vi "HFRR ADV v025 new software.vi"() -> ()   [LabVIEW 2025] (continued)
            n902 = call <vilib>:"Trim Whitespace.vi"("string"="C:\\LAB-IQ\\images\\") -> ("trimmed string"=w1151:string)  [unwired: 1 in]
            n903 = String To Path(string=w1151) -> (path=w1150:path)
            n904 = Concatenate Strings(w1149, ".png" ("string")) -> (w1148:string)
            n905 = Build Path(base path=w1150, name or relative path=w1148) -> (appended path=w1146:path)
            n906 = Path To String(path=w1146) -> (string=w1145:string)
            n907 = call "CAMERA LIVE FEED FGV.vi"("Enum - Menu"=CAMERA_LIVE_FEED_ENUM."CAMERA SAVE", "Image Path"=w1145) -> ("error out"=w1143:errorcluster)  [unwired: 8 in, 1 out]
            n908 = case shown="No Error" w1143 {
              frame No Error {
                n909 = One Button Dialog(message="Image saved successfully") -> ()  [unwired: 1 in, 1 out]
              }
              frame Error {
              }
            }
          }
          frame #3 {
            n910 = call "LIST FILE NAMES.vi"() -> ("error out"=w1157:errorcluster, "filenames"=w1154:string[])  [unwired: 10 in]
            n911 = call "IMAGE ANALYSIS.vi"("Enum"=POST_ANALYSIS_ENUM."SHOW UI", "error in"=w1157) -> ("error out"=w1155:errorcluster)  [unwired: 8 in, 1 out]
            n912 = property on="Test File List :" class="CmbBox"("Strings[]"=w1154) -> ()  [unwired: 2 in, 2 out]
          }
          frame #4 {
            (unwired) T22."Report" ("Main Dashboard Buttons")
            (unwired) T24."Report" ("Main Dashboard Buttons")
            n913 = Not(x=w1162) -> (.not. x?=w1161:bool)
            n914 = local write "Zoom Factore"(0.0 ("Zoom Factore")) -> ()
            n915 = local write "Cap Live Image"(w1161) -> ()
            n916 = local write "Main Tab"(T2."Adv Scar Report" ("Main Tab")) -> ()
            n917 = property on="Cap Live Image" class="Bool (strict)"("BoolText.Text"="Capture Image" ("Boolean Text.Text")) -> ()  [unwired: 2 in, 2 out]
            n918 = local write "Main Dashboard Buttons"(T1."Report" ("Main Dashboard Buttons")) -> ()
          }
        }
      }
    }
    n919 = local read "change Gain"() -> (w808:bool)
    n920 = local read "Back Square"() -> (w807:bool)
    n921 = case shown="True" w808 {
      selector: w808 -> [_ w852]
      frame False {
      }
      frame True {
        n922 = stacked-sequence {
          tunnel: w852 -> [_ w860]
          frame #0 {
            n923 = local read "Actual (µm)"() -> (w856:dbl)
            n924 = local read "Pixel Value"() -> (w855:dbl)
            n925 = local read "Magnification :"() -> (w854:string)
            n926 = Divide(x=w856, y=w855) -> (x/y=w853:dbl)
            n927 = case shown="\"10x\"" w854 {
              tunnel: w853 -> [w857 w858]
              frame "10x" {
                n928 = local write "10x Gain"(w857) -> ()
              }
              frame "5x", Default {
                n929 = local write "5x Gain"(w858) -> ()
              }
            }
          }
          frame #1 {
            n930 = Not(x=w860) -> (.not. x?=w859:bool)
            n931 = local write "change Gain"(w859) -> ()
          }
        }
      }
    }
    n932 = case shown="True" w807 {
      selector: w807 -> [_ w850]
      frame False {
      }
      frame True {
        n933 = Not(x=w850) -> (.not. x?=w849:bool)
        n934 = local write "Back Square"(w849) -> ()
        n935 = local write "Calibration Tab"(enum32{"Measrument", "Calibrate"}."Measrument" ("Calibration Tab")) -> ()
      }
    }
    n936 = local read "Rectangle Tool"() -> (w819:bool)
    n937 = local read "Clear ROI Tool"() -> (w818:bool)
    n938 = local read "Open Image"() -> (w823:bool)
    n939 = local read "line tool"() -> (w820:bool)
    n940 = local read "OUT"() -> (w821:bool)
    n941 = local read "In"() -> (w822:bool)
    n942 = case shown="True" w823 {
      selector: w823 -> [_ w1128]
      tunnel: [w1124 w1130] -> _
      tunnel: w813 -> [w1124 w1129]
      frame False {
      }
      frame True {
        n943 = Not(x=w1128) -> (.not. x?=w1127:bool)
        n944 = local write "Open Image"(w1127) -> ()
        n945 = call "IMAGE ANALYSIS.vi"("Enum"=POST_ANALYSIS_ENUM."HIDE UI", "error in"=w1129) -> ("error out"=w1137:errorcluster)  [unwired: 8 in, 1 out]
        n946 = call "File Dialog"("start path"=path "C:/LAB-IQ/images", "error in"=w1137) -> ("selected path"=w1126:path, "error out"=w1135:errorcluster)  [unwired: 10 in, 2 out]
        "Image path  2" <- w1126
        n947 = call <vilib>:"Clear Errors.vi"("error in (no error)"=w1135) -> ("error out"=w1134:errorcluster)  [unwired: 5 in, 1 out]
        n948 = call "IMAGE ANALYSIS.vi"("Enum"=POST_ANALYSIS_ENUM."OPEN FILE", "error in"=w1134, "File Path"=w1126) -> ("error out"=w1133:errorcluster)  [unwired: 7 in, 1 out]
        n949 = call <vilib>:"Clear Errors.vi"("error in (no error)"=w1133) -> ("error out"=w1132:errorcluster)  [unwired: 5 in, 1 out]
        n950 = call "IMAGE ANALYSIS.vi"("Enum"=POST_ANALYSIS_ENUM."SHOW UI", "error in"=w1132) -> ("error out"=w1130:errorcluster)  [unwired: 8 in, 1 out]
        n951 = local write "Zoom Factore"(100.0 ("Zoom Factore")) -> ()
      }
    }
    n952 = case shown="True" w821 {
      selector: w821 -> [_ w1109]
      tunnel: w813 -> [w1106 w1114]
      tunnel: [w1106 w1108] -> _
      frame False {
      }
      frame True {
        n953 = Not(x=w1109) -> (.not. x?=w1107:bool)
        n954 = local read "Zoom Factore"() -> (w1112:dbl)
        n955 = local write "OUT"(w1107) -> ()
        n956 = call "IMAGE ANALYSIS.vi"("Enum"=POST_ANALYSIS_ENUM."ZOOM OUT", "error in"=w1114) -> ("error out"=w1108:errorcluster)  [unwired: 8 in, 1 out]
        n957 = Divide(x=w1112, y=1.2) -> (x/y=w1110:dbl)
        n958 = local write "Zoom Factore"(w1110) -> ()
      }
    }
    n959 = case shown="True" w822 {
      selector: w822 -> [_ w1118]
      tunnel: w813 -> [w1115 w1123]
      tunnel: [w1115 w1116] -> _
      frame False {
      }
      frame True {
        n960 = Not(x=w1118) -> (.not. x?=w1117:bool)
        n961 = local read "Zoom Factore"() -> (w1121:dbl)
        n962 = local write "In"(w1117) -> ()
        n963 = call "IMAGE ANALYSIS.vi"("Enum"=POST_ANALYSIS_ENUM."ZOOM IN", "error in"=w1123) -> ("error out"=w1116:errorcluster)  [unwired: 8 in, 1 out]
        n964 = Multiply(x=w1121, y=1.2) -> (x*y=w1119:dbl)
        n965 = local write "Zoom Factore"(w1119) -> ()
      }
    }
    n966 = case shown="True" w818 {
      selector: w818 -> [_ w1090]
      tunnel: w813 -> [w1088 w1092]
      tunnel: [w1088 w1091] -> _
      frame False {
      }
      frame True {
        n967 = Not(x=w1090) -> (.not. x?=w1089:bool)
        n968 = local write "Clear ROI Tool"(w1089) -> ()
        n969 = call "IMAGE ANALYSIS.vi"("Enum"=POST_ANALYSIS_ENUM."CLEAR ROI", "error in"=w1092) -> ("error out"=w1091:errorcluster)  [unwired: 8 in, 1 out]
      }
    }
    n970 = case shown="True" w820 {
      selector: w820 -> [_ w1102]
      tunnel: w813 -> [w1100 w1105]
      tunnel: [w1100 w1103] -> _
      frame False {
      }
      frame True {
        n971 = Not(x=w1102) -> (.not. x?=w1101:bool)
        n972 = local write "line tool"(w1101) -> ()
        n973 = call "IMAGE ANALYSIS.vi"("Enum"=POST_ANALYSIS_ENUM."DRAW LINE", "error in"=w1105) -> ("error out"=w1103:errorcluster)  [unwired: 8 in, 1 out]
      }
    }
    n974 = case shown="True" w819 {
      selector: w819 -> [_ w1096]
      tunnel: w813 -> [w1094 w1098]
      tunnel: [w1094 w1097] -> _
      frame False {
      }
      frame True {
        n975 = Not(x=w1096) -> (.not. x?=w1095:bool)
        n976 = local write "Rectangle Tool"(w1095) -> ()
        n977 = call "IMAGE ANALYSIS.vi"("Enum"=POST_ANALYSIS_ENUM."DRAW REC", "error in"=w1098) -> ("error out"=w1097:errorcluster)  [unwired: 8 in, 1 out]
      }
    }
    n978 = local read "SCAR MEASURMENT"() -> (w806:enum32{"Auto Scar", "Manual Scar"})
    n979 = local read "Fit to Screen Tool"() -> (w815:bool)
    n980 = local read "Resize Tool"() -> (w814:bool)
    n981 = case shown="\"Manual Scar\", Default" w806 {
      frame "Auto Scar" {
        n982 = property on="Cap Live Image" class="Bool (strict)"("BoolText.Text"="Report" ("Boolean Text.Text")) -> ()  [unwired: 2 in, 2 out]
      }
      frame "Manual Scar", Default {
        n983 = property on="Cap Live Image" class="Bool (strict)"("BoolText.Text"="Save Image" ("Boolean Text.Text")) -> ()  [unwired: 2 in, 2 out]
      }
    }
    n984 = local read "ROI Color Tool"() -> (w816:bool)
    n985 = local read "Pan Tool"() -> (w817:bool)
    n986 = case shown="True" w817 {
      selector: w817 -> [_ w1084]
      tunnel: w813 -> [w1082 w1086]
      tunnel: [w1082 w1085] -> _
      frame False {
      }
      frame True {
        n987 = Not(x=w1084) -> (.not. x?=w1083:bool)
        n988 = call "IMAGE ANALYSIS.vi"("Enum"=POST_ANALYSIS_ENUM."PAN", "error in"=w1086) -> ("error out"=w1085:errorcluster)  [unwired: 8 in, 1 out]
        n989 = local write "Pan Tool"(w1083) -> ()
      }
    }
    n990 = case shown="True" w814 {
      selector: w814 -> [_ w1068]
      tunnel: w813 -> [w1063 w1065]
      tunnel: [w1063 w1064] -> _
      frame False {
      }
      frame True {
        n991 = Not(x=w1068) -> (.not. x?=w1067:bool)
        n992 = local write "Resize Tool"(w1067) -> ()
        n993 = call "IMAGE ANALYSIS.vi"("Enum"=POST_ANALYSIS_ENUM."RESIZE MODE", "error in"=w1065) -> ("error out"=w1064:errorcluster)  [unwired: 8 in, 1 out]
      }
    }
    n994 = case shown="True" w815 {
      selector: w815 -> [_ w1073]
      tunnel: [w1069 w1074] -> _
      tunnel: w813 -> [w1069 w1072]
      frame False {
      }
      frame True {
        n995 = Not(x=w1073) -> (.not. x?=w1071:bool)
        n996 = local write "Zoom Factore"(100.0 ("Zoom Factore")) -> ()
        n997 = local write "Fit to Screen Tool"(w1071) -> ()
        n998 = call "IMAGE ANALYSIS.vi"("Enum"=POST_ANALYSIS_ENUM."FIT", "error in"=w1072) -> ("error out"=w1074:errorcluster)  [unwired: 8 in, 1 out]
      }
    }
    n999 = case shown="True" w816 {
      selector: w816 -> [_ w1079]
      tunnel: [w1076 w1080] -> _
      tunnel: w813 -> [w1076 w1077]
      frame False {
      }
      frame True {
        n1000 = Not(x=w1079) -> (.not. x?=w1078:bool)
        n1001 = local write "ROI Color Tool"(w1078) -> ()
        n1002 = call "IMAGE ANALYSIS.vi"("Enum"=POST_ANALYSIS_ENUM."SET ROI COLOR", "error in"=w1077) -> ("error out"=w1080:errorcluster)  [unwired: 8 in, 1 out]
      }
    }
    n1003 = local read "Quit"() -> (w830:bool)
  }
  n1004 = while {
    stop <- w1164 stop-if-true
    n1005 = local read "Image Path"() -> (w1167:path)
    n1006 = local read "Print 3"() -> (w1170:bool)
    n1007 = Equal?(x=w1167, y=path "") -> (x = y?=w1166:bool)
    n1008 = Not(x=w1166) -> (.not. x?=w1165:bool)
    n1009 = property on="Print 3" class="Bool (strict)"("Visible"=w1165) -> ()  [unwired: 2 in, 2 out]
    n1010 = case shown="True" w1170 {
      frame False {
        n1011 = local write "Rd"(TRUE ("Boolean 7")) -> ()
      }
      frame True {
        n1012 = flat-sequence {
          tunnel: [w1210] -> w1178
          tunnel: [w1197] -> w1176
          tunnel: [w1207] -> w1172
          tunnel: w1178 -> [w1219]
          tunnel: [w1219] -> w1177
          tunnel: w1176 -> [w1218]
          tunnel: [w1218] -> w1175
          tunnel: [w1216] -> w1174
          tunnel: [w1215] -> w1173
          tunnel: w1172 -> [w1215]
          tunnel: w1177 -> [w1221]
          tunnel: w1175 -> [w1222]
          tunnel: w1174 -> [_]
          tunnel: w1173 -> [w1220]
          frame #0 {
            n1013 = case shown="True" "Rd" {
              frame False {
              }
              frame True {
                n1014 = while {
                  tunnel: "abcdefABCDEF" ("string 2") -> [w1189]
                  shift-right: [w1187] -> w1181
                  shift-left: "" -> [w1186]
                  i -> [w1196]
                  stop <- w1195 stop-if-true
                  n1015 = Random Number (0-1)() -> (number: 0 to 1=w1190:dbl)
                  n1016 = Multiply(x=w1190, y=62.0) -> (x*y=w1192:dbl)
                  n1017 = Decrement(x="Length 2") -> (x-1=w1185:i16)
                  n1018 = To Word Integer(number=w1192) -> (16bit integer=w1193:i16)
                  n1019 = String Subset(string=w1189, offset (0)=w1193, length (rest)=1 ("length (rest)")) -> (substring=w1188:string)
                  n1020 = Greater Or Equal?(x=w1196, y=w1185) -> (x >= y?=w1195:bool)
                  n1021 = Concatenate Strings(w1188, w1186) -> (w1187:string)
                }
                "String 10" <- w1181
                n1022 = local write "Rd"(FALSE ("Boolean 7")) -> ()
              }
            }
          }
          frame #1 {
            w1208 = "_resized.jpg" ("command line")
            (unwired) ".jpg -resize 320x240 " ("string")
            (unwired) "Choose an Image File" ("prompt")
            # "-resize 1798x425"
            n1023 = local read "Image Path"() -> (w1202:path)
            n1024 = Strip Path(path=w1202) -> (stripped path=w1197:path, name=w1198:string)
            n1025 = Match Pattern(string=w1198, regular expression=".jpg") -> (before substring=→"before substring 2":string, after substring=→"after substring":string)  [unwired: 1 in, 2 out]
            n1026 = Match Pattern(string=w1198, regular expression="\\") -> (before substring=w1204:string)  [unwired: 1 in, 3 out]
            n1027 = Match Pattern(string=w1204, regular expression=".jpg") -> (before substring=w1203:string)  [unwired: 1 in, 3 out]
            n1028 = Concatenate Strings("cmd /c convert " ("string"), w1203, ".jpg -resize 320x240  " ("command line"), w1203, w1208) -> (w1211:string)
            n1029 = call <vilib>:"System Exec.vi"("run minimized? (F)"=TRUE, "wait until completion? (T)"=TRUE, "working directory"=w1197, "command line"=w1211) -> ("error out"=w1210:errorcluster)  [unwired: 4 in, 3 out]
            "error out 2" <- w1210
            n1030 = Concatenate Strings(w1203, w1208) -> (w1207:string)
          }
          frame #2 {
            n1031 = Wait (ms)(milliseconds to wait=u32 2000 ("millisecond timer value")) -> (millisecond timer value=w1216:u32)
          }
          frame #3 {
            n1032 = case shown="No Error" w1221 {
              tunnel: w1222 -> [w1225 _]
              tunnel: w1220 -> [w1223 _]
              frame No Error {
                (unwired) ".jpg" ("string")
                n1033 = Path To String(path=w1225) -> (string=w1229:string)
                n1034 = Concatenate Strings(w1229, "\\" ("string"), w1223) -> (w1228:string)
                n1035 = String To Path(string=w1228) -> (path=w1227:path)
                n1036 = call <vilib>:"Read JPEG File.vi"("path to JPEG file"=w1227) -> ("image data"=w1231:T14)  [unwired: 8 in, 2 out]
                "image data" <- w1231
                n1037 = local write "Print 3"(FALSE ("Print 2")) -> ()
                n1038 = call <vilib>:"Draw Flattened Pixmap.vi"("image data"=w1231) -> ("new picture"=→"new picture":picture)  [unwired: 8 in]
              }
              frame Error {
              }
            }
          }
        }
      }
    }
    n1039 = Wait (ms)(milliseconds to wait=u32 20 ("millisecond timer value")) -> ()  [unwired: 1 out]
    n1040 = local read "Quit"() -> (w1164:bool)
  }
  n1041 = while {
    tunnel: w38 -> [_]
    tunnel: w24 -> [_]
    stop <- w1262 stop-if-true
    # "New Adv Logics"
    n1042 = local read "Main Tab"() -> (w1242:T2)
    n1043 = local read "Main Tab"() -> (w1260:T2)
    n1044 = local read "Sign In"() -> (w1259:bool)
    n1045 = case shown="\"Adv Scar\"" w1242 {
      frame "HOME", Default {
        n1046 = local read "LIVE FEED MIN TEMP"() -> (w1395:bool)
        n1047 = local write "LIVE FEED MAX TEMP"(TRUE ("LIVE FEED MAX TEMP")) -> ()
        n1048 = local read "CAMERA ROI MIN TEMP"() -> (w1393:bool)
        n1049 = case shown="True" w1395 {
          selector: w1395 -> [_ w1402]
          frame False {
          }
          frame True {
            n1050 = Not(x=w1402) -> (.not. x?=w1401:bool)
            n1051 = local write "LIVE FEED MIN TEMP"(w1401) -> ()
            n1052 = call "CAMERA LIVE FEED FGV.vi"("Enum - Menu"=CAMERA_LIVE_FEED_ENUM."CAMERA MINIMIZE") -> ()  [unwired: 9 in, 2 out]
          }
        }
        n1053 = case shown="True" w1393 {
          selector: w1393 -> [_ w1399]
          frame False {
          }
          frame True {
            n1054 = Not(x=w1399) -> (.not. x?=w1398:bool)
            n1055 = local write "CAMERA ROI MIN TEMP"(w1398) -> ()
            n1056 = call "IMAGE ANALYSIS.vi"("Enum"=POST_ANALYSIS_ENUM."MINIMIZE UI") -> ()  [unwired: 9 in, 2 out]
          }
        }
        n1057 = local write "CAMERA ROI MAX TEMP"(TRUE ("CAMERA ROI MAX TEMP")) -> ()
      }
      frame "Test Setup" {
        n1058 = local read "LIVE FEED MIN TEMP"() -> (w1405:bool)
        n1059 = local read "CAMERA ROI MIN TEMP"() -> (w1403:bool)
        n1060 = local write "LIVE FEED MAX TEMP"(TRUE ("LIVE FEED MAX TEMP")) -> ()
        n1061 = case shown="True" w1405 {
          selector: w1405 -> [_ w1412]
          frame False {
          }
          frame True {
            n1062 = Not(x=w1412) -> (.not. x?=w1411:bool)
            n1063 = local write "LIVE FEED MIN TEMP"(w1411) -> ()
            n1064 = call "CAMERA LIVE FEED FGV.vi"("Enum - Menu"=CAMERA_LIVE_FEED_ENUM."CAMERA MINIMIZE") -> ()  [unwired: 9 in, 2 out]
          }
        }
        n1065 = case shown="True" w1403 {
          selector: w1403 -> [_ w1409]
          frame False {
          }
          frame True {
            n1066 = Not(x=w1409) -> (.not. x?=w1408:bool)
            n1067 = local write "CAMERA ROI MIN TEMP"(w1408) -> ()
            n1068 = call "IMAGE ANALYSIS.vi"("Enum"=POST_ANALYSIS_ENUM."MINIMIZE UI") -> ()  [unwired: 9 in, 2 out]
          }
        }
        n1069 = local write "CAMERA ROI MAX TEMP"(TRUE ("CAMERA ROI MAX TEMP")) -> ()
      }
      frame "Acquire" {
        n1070 = local read "LIVE FEED MIN TEMP"() -> (w1415:bool)
        n1071 = local write "LIVE FEED MAX TEMP"(TRUE ("LIVE FEED MAX TEMP")) -> ()
        n1072 = local read "CAMERA ROI MIN TEMP"() -> (w1413:bool)
        n1073 = case shown="True" w1415 {
          selector: w1415 -> [_ w1422]
          frame False {
          }
          frame True {
            n1074 = Not(x=w1422) -> (.not. x?=w1421:bool)
            n1075 = local write "LIVE FEED MIN TEMP"(w1421) -> ()
            n1076 = call "CAMERA LIVE FEED FGV.vi"("Enum - Menu"=CAMERA_LIVE_FEED_ENUM."CAMERA MINIMIZE") -> ()  [unwired: 9 in, 2 out]
          }
        }
        n1077 = case shown="True" w1413 {
          selector: w1413 -> [_ w1419]
          frame False {
          }
          frame True {
            n1078 = Not(x=w1419) -> (.not. x?=w1418:bool)
            n1079 = local write "CAMERA ROI MIN TEMP"(w1418) -> ()
            n1080 = call "IMAGE ANALYSIS.vi"("Enum"=POST_ANALYSIS_ENUM."MINIMIZE UI") -> ()  [unwired: 9 in, 2 out]
          }
        }
        n1081 = local write "CAMERA ROI MAX TEMP"(TRUE ("CAMERA ROI MAX TEMP")) -> ()
      }
      frame "Adv Scar" {
        n1082 = local read "CAMERA ROI MIN TEMP"() -> (w1423:bool)
        n1083 = case shown="True" "LIVE FEED MAX TEMP" {
          selector: "LIVE FEED MAX TEMP" -> [_ w1444]
          frame False {
          }
          frame True {
            n1084 = Not(x=w1444) -> (.not. x?=w1443:bool)
            n1085 = local write "LIVE FEED MAX TEMP"(w1443) -> ()
            n1086 = call "CAMERA LIVE FEED FGV.vi"("Enum - Menu"=CAMERA_LIVE_FEED_ENUM."CAMERA RESTORE") -> ("error out"=w1434:errorcluster)  [unwired: 9 in, 1 out]
            n1087 = Type Cast(type=30, x=0) -> (*(type *) &x=w1438:i32)
            n1088 = Add(x=w1438, y=48) -> (x+y=w1439:i32)
            n1089 = call "CAMERA LIVE FEED FGV.vi"("Enum - Menu"=CAMERA_LIVE_FEED_ENUM."CAMERA MODE SET", "error in (no error)"=w1434, "CAMERA MODE"=w1439) -> ("error out"=w1431:errorcluster)  [unwired: 7 in, 1 out]
            n1090 = call "CAMERA LIVE FEED FGV.vi"("Enum - Menu"=CAMERA_LIVE_FEED_ENUM."CAMERA GRAY", "error in (no error)"=w1431) -> ("error out"=w1430:errorcluster)  [unwired: 8 in, 1 out]
            n1091 = call "LIST FILE NAMES.vi"("error in (no error)"=w1430) -> ("error out"=w1440:errorcluster, "filenames"=w1441:string[])  [unwired: 9 in]
            n1092 = property on="FILE 3" class="CmbBox"(error in=w1440, "Strings[]"=w1441) -> ()  [unwired: 1 in, 2 out]
          }
        }
        n1093 = case shown="True" w1423 {
          selector: w1423 -> [_ w1429]
          frame False {
          }
          frame True {
            n1094 = Not(x=w1429) -> (.not. x?=w1428:bool)
            n1095 = local write "CAMERA ROI MIN TEMP"(w1428) -> ()
            n1096 = call "IMAGE ANALYSIS.vi"("Enum"=POST_ANALYSIS_ENUM."MINIMIZE UI") -> ()  [unwired: 9 in, 2 out]
          }
        }
        n1097 = local write "CAMERA ROI MAX TEMP"(TRUE ("CAMERA ROI MAX TEMP")) -> ()
        "LIVE FEED MIN TEMP" <- TRUE ("LIVE FEED MIN TEMP")
      }
      frame "Adv Scar Report" {
        n1098 = local read "CAMERA ROI MAX TEMP"() -> (w1445:bool)
        n1099 = local read "LIVE FEED MIN TEMP"() -> (w1447:bool)
        n1100 = local write "LIVE FEED MAX TEMP"(TRUE ("LIVE FEED MAX TEMP")) -> ()
        n1101 = case shown="True" w1447 {
          selector: w1447 -> [_ w1456]
          frame False {
          }
          frame True {
            n1102 = Not(x=w1456) -> (.not. x?=w1455:bool)
            n1103 = local write "LIVE FEED MIN TEMP"(w1455) -> ()
            n1104 = call "CAMERA LIVE FEED FGV.vi"("Enum - Menu"=CAMERA_LIVE_FEED_ENUM."CAMERA MINIMIZE") -> ()  [unwired: 9 in, 2 out]
          }
        }
        n1105 = case shown="True" w1445 {
          selector: w1445 -> [_ w1453]
          frame False {
          }
          frame True {
            n1106 = Not(x=w1453) -> (.not. x?=w1451:bool)
            n1107 = local write "CAMERA ROI MAX TEMP"(w1451) -> ()
            n1108 = call "IMAGE ANALYSIS.vi"("Enum"=POST_ANALYSIS_ENUM."SHOW UI") -> ("error out"=w1450:errorcluster)  [unwired: 9 in, 1 out]
            n1109 = call "LIST FILE NAMES.vi"("error in (no error)"=w1450) -> ("filenames"=w1449:string[])  [unwired: 9 in, 1 out]
            n1110 = property on="Test File List :" class="CmbBox"("Strings[]"=w1449) -> ()  [unwired: 2 in, 2 out]
          }
        }
        n1111 = local write "CAMERA ROI MIN TEMP"(TRUE ("CAMERA ROI MIN TEMP")) -> ()
      }
      frame "Compare Files" {
        n1112 = local read "LIVE FEED MIN TEMP"() -> (w1459:bool)
        n1113 = local write "LIVE FEED MAX TEMP"(TRUE ("LIVE FEED MAX TEMP")) -> ()
        n1114 = local read "CAMERA ROI MIN TEMP"() -> (w1457:bool)
        n1115 = case shown="True" w1459 {
          selector: w1459 -> [_ w1466]
          frame False {
          }
          frame True {
            n1116 = Not(x=w1466) -> (.not. x?=w1465:bool)
            n1117 = local write "LIVE FEED MIN TEMP"(w1465) -> ()
            n1118 = call "CAMERA LIVE FEED FGV.vi"("Enum - Menu"=CAMERA_LIVE_FEED_ENUM."CAMERA MINIMIZE") -> ()  [unwired: 9 in, 2 out]
          }
        }
        n1119 = case shown="True" w1457 {
          selector: w1457 -> [_ w1463]
          frame False {
          }
          frame True {
            n1120 = Not(x=w1463) -> (.not. x?=w1462:bool)
            n1121 = local write "CAMERA ROI MIN TEMP"(w1462) -> ()
            n1122 = call "IMAGE ANALYSIS.vi"("Enum"=POST_ANALYSIS_ENUM."MINIMIZE UI") -> ()  [unwired: 9 in, 2 out]
          }
        }
        n1123 = local write "CAMERA ROI MAX TEMP"(TRUE ("CAMERA ROI MAX TEMP")) -> ()
      }
      frame "About" {
        n1124 = local read "LIVE FEED MIN TEMP"() -> (w1469:bool)
        n1125 = local write "LIVE FEED MAX TEMP"(TRUE ("LIVE FEED MAX TEMP")) -> ()
        n1126 = local read "CAMERA ROI MIN TEMP"() -> (w1468:bool)
        n1127 = case shown="True" w1469 {
          selector: w1469 -> [_ w1476]
          frame False {
          }
          frame True {
            n1128 = Not(x=w1476) -> (.not. x?=w1475:bool)
            n1129 = local write "LIVE FEED MIN TEMP"(w1475) -> ()
            n1130 = call "CAMERA LIVE FEED FGV.vi"("Enum - Menu"=CAMERA_LIVE_FEED_ENUM."CAMERA MINIMIZE") -> ()  [unwired: 9 in, 2 out]
          }
        }
        n1131 = case shown="True" w1468 {
          selector: w1468 -> [_ w1473]
          frame False {
          }
          frame True {
            n1132 = Not(x=w1473) -> (.not. x?=w1472:bool)
            n1133 = local write "CAMERA ROI MIN TEMP"(w1472) -> ()
            n1134 = call "IMAGE ANALYSIS.vi"("Enum"=POST_ANALYSIS_ENUM."MINIMIZE UI") -> ()  [unwired: 9 in, 2 out]
          }
        }
        n1135 = local write "CAMERA ROI MAX TEMP"(TRUE ("CAMERA ROI MIN TEMP")) -> ()
      }
      frame "Advance" {
        n1136 = local read "LIVE FEED MIN TEMP"() -> (w1479:bool)
        n1137 = local write "LIVE FEED MAX TEMP"(TRUE ("LIVE FEED MAX TEMP")) -> ()
        n1138 = local read "CAMERA ROI MIN TEMP"() -> (w1477:bool)
        n1139 = case shown="True" w1479 {
          selector: w1479 -> [_ w1486]
          frame False {
          }
          frame True {
            n1140 = Not(x=w1486) -> (.not. x?=w1485:bool)
            n1141 = local write "LIVE FEED MIN TEMP"(w1485) -> ()
            n1142 = call "CAMERA LIVE FEED FGV.vi"("Enum - Menu"=CAMERA_LIVE_FEED_ENUM."CAMERA MINIMIZE") -> ()  [unwired: 9 in, 2 out]
          }
        }
        n1143 = local write "CAMERA ROI MAX TEMP"(TRUE ("CAMERA ROI MAX TEMP")) -> ()
        n1144 = case shown="True" w1477 {
          selector: w1477 -> [_ w1483]
          frame False {
          }
          frame True {
            n1145 = Not(x=w1483) -> (.not. x?=w1482:bool)
            n1146 = local write "CAMERA ROI MIN TEMP"(w1482) -> ()
            n1147 = call "IMAGE ANALYSIS.vi"("Enum"=POST_ANALYSIS_ENUM."MINIMIZE UI") -> ()  [unwired: 9 in, 2 out]
          }
        }
      }
      frame "Mooha" {
        n1148 = local read "LIVE FEED MIN TEMP"() -> (w1489:bool)
        n1149 = local write "LIVE FEED MAX TEMP"(TRUE ("LIVE FEED MAX TEMP")) -> ()
        n1150 = local read "CAMERA ROI MIN TEMP"() -> (w1487:bool)
        n1151 = case shown="True" w1489 {
          selector: w1489 -> [_ w1496]
          frame False {
          }
          frame True {
            n1152 = Not(x=w1496) -> (.not. x?=w1495:bool)
            n1153 = local write "LIVE FEED MIN TEMP"(w1495) -> ()
            n1154 = call "CAMERA LIVE FEED FGV.vi"("Enum - Menu"=CAMERA_LIVE_FEED_ENUM."CAMERA MINIMIZE") -> ()  [unwired: 9 in, 2 out]
          }
        }
        n1155 = local write "CAMERA ROI MAX TEMP"(TRUE ("CAMERA ROI MAX TEMP")) -> ()
        n1156 = case shown="True" w1487 {
          selector: w1487 -> [_ w1493]
          frame False {
          }
          frame True {
            n1157 = Not(x=w1493) -> (.not. x?=w1492:bool)
            n1158 = local write "CAMERA ROI MIN TEMP"(w1492) -> ()
            n1159 = call "IMAGE ANALYSIS.vi"("Enum"=POST_ANALYSIS_ENUM."MINIMIZE UI") -> ()  [unwired: 9 in, 2 out]
          }
        }
      }
    }
    n1160 = local read "Auto Start Test"() -> (w1233:bool)
    n1161 = case shown="True" "sign in temp" {
      frame False {
      }
      frame True {
        w1269 = 1 ("y")
        n1162 = local read "USERNAME"() -> (w1275:string)
        n1163 = local read "USER ID"() -> (w1272:string)
        n1164 = call <vilib>:"Trim Whitespace.vi"("string"=w1275) -> ("trimmed string"=w1274:string)  [unwired: 1 in]
        n1165 = call <vilib>:"Trim Whitespace.vi"("string"=w1272) -> ("trimmed string"=w1273:string)  [unwired: 1 in]
        n1166 = String Length(string=w1274) -> (length=w1271:i32)
        n1167 = String Length(string=w1273) -> (length=w1270:i32)
        n1168 = Greater?(x=w1271, y=w1269) -> (0:w1268:bool)
        n1169 = Greater?(x=w1270, y=w1269) -> (0:w1267:bool)
        n1170 = And(x=w1268, y=w1267) -> (x .and. y?=w1266:bool)
        n1171 = case shown="True" w1266 {
          frame False {
            n1172 = property on="Sign In" class="Bool (strict)"("DisabledEnum"=T17."Disabled" ("Disabled")) -> ()  [unwired: 2 in, 2 out]
          }
          frame True {
            n1173 = property on="Sign In" class="Bool (strict)"("DisabledEnum"=T17."Enabled" ("Disabled")) -> ()  [unwired: 2 in, 2 out]
          }
        }
      }
    }
    n1174 = local read "Air Temperature"() -> (w1250:bool)
    n1175 = local read "Coefficient Of Friction"() -> (w1251:bool)
    n1176 = case shown="False" w1233 {
      frame False {
        n1177 = local read "Auto stop temp"() -> (w1263:bool)
        n1178 = case shown="True" w1263 {
          frame False {
          }
          frame True {
            n1179 = local write "Auto Start Temp"(FALSE ("Auto Start Temp")) -> ()
          }
        }
      }
      frame True {
        "Auto stop temp" <- TRUE ("Auto stop temp")
      }
    }
    n1180 = local read "Humidity"() -> (w1249:bool)
    n1181 = case shown="\"HOME\"" w1260 {
      frame "HOME" {
        n1182 = local write "main tab sub"(enum32{"Page 1", "Page 2"}."Page 1" ("main tab sub")) -> ()
      }
      frame Default {
        n1183 = local write "main tab sub"(enum32{"Page 1", "Page 2"}."Page 2" ("main tab sub")) -> ()
      }
    }
    n1184 = case shown="True" w1259 {
      selector: w1259 -> [_ w1610]
      frame False {
      }
      frame True {
        n1185 = Not(x=w1610) -> (.not. x?=w1609:bool)
        n1186 = local write "Sign In"(w1609) -> ()
        n1187 = local write "Main Dashboard Buttons"(T22."Test Setup" ("Main Dashboard Buttons")) -> ()
      }
    }
    n1188 = case shown="\"Numeric Display\", Default" "Num/Graph" {
      frame "Numeric Display", Default {
        n1189 = property on="Single/Multiple" class="RadioBtnsControl (strict)"("Visible"=FALSE) -> ()  [unwired: 2 in, 2 out]
        n1190 = property on="Single - Graph" class="Ring (strict)"("Visible"=FALSE) -> ()  [unwired: 2 in, 2 out]
        n1191 = local write "Main Tab Display"(T4."Dashboard 1" ("Main Tab Display")) -> ()
      }
      frame "Graph Display" {
        n1192 = property on="Single/Multiple" class="RadioBtnsControl (strict)"("Visible"=TRUE) -> ()  [unwired: 2 in, 2 out]
        n1193 = case shown="\"Multiple\"" "Single/Multiple" {
          frame "Single ", Default {
            n1194 = property on="Single - Graph" class="Ring (strict)"("Visible"=TRUE) -> ()  [unwired: 2 in, 2 out]
            n1195 = local write "Main Tab Display"(T4."Dashboard 3" ("Main Tab Display")) -> ()
          }
          frame "Multiple" {
            n1196 = property on="Single - Graph" class="Ring (strict)"("Visible"=FALSE) -> ()  [unwired: 2 in, 2 out]
            n1197 = local write "Main Tab Display"(T4."Dashboard 2" ("Main Tab Display")) -> ()
          }
        }
      }
    }
    n1198 = local read "Stroke"() -> (w1248:bool)
    n1199 = local read "USERNAME"() -> (w1254:string)
    n1200 = local read "USER ID"() -> (w1253:string)
    n1201 = case shown="True" w1251 {
      selector: w1251 -> [_ w1536]
      frame False {
      }
      frame True {
        n1202 = Not(x=w1536) -> (.not. x?=w1535:bool)
        n1203 = local write "Coefficient Of Friction"(w1535) -> ()
        n1204 = local write "Tab Control 2"(T6."Coefficient Of Friction" ("Tab Control 2")) -> ()
      }
    }
    n1205 = case shown="True" w1250 {
      selector: w1250 -> [_ w1533]
      frame False {
      }
      frame True {
        n1206 = Not(x=w1533) -> (.not. x?=w1531:bool)
        n1207 = local write "Air Temperature"(w1531) -> ()
        n1208 = local write "Tab Control 2"(T6."Air Temperature" ("Tab Control 2")) -> ()
      }
    }
    n1209 = local write "Operator ID"(w1253) -> ()
    n1210 = case shown="True" w1248 {
      selector: w1248 -> [_ w1527]
      frame False {
      }
      frame True {
        n1211 = Not(x=w1527) -> (.not. x?=w1525:bool)
        n1212 = local write "Stroke"(w1525) -> ()
        n1213 = local write "Tab Control 2"(T6."Stroke" ("Tab Control 2")) -> ()
      }
    }
    n1214 = local write "tested by"(w1254) -> ()
    n1215 = case shown="True" w1249 {
      selector: w1249 -> [_ w1530]
      frame False {
      }
      frame True {
        n1216 = Not(x=w1530) -> (.not. x?=w1528:bool)
        n1217 = local write "Humidity"(w1528) -> ()
        n1218 = local write "Tab Control 2"(T6."Humidity" ("Tab Control 2")) -> ()
      }
    }
    n1219 = case shown="\"Calibration\"" "Main Dashboard Buttons" {
      tunnel: [T2."HOME" ("Main Tab") T2."Test Setup" ("Main Tab") T2."Acquire" ("Main Tab") T2."Adv Scar" ("Main Tab") T2."Adv Scar Report" ("Main Tab") T2."Compare Files" ("Main Tab") T2."Calibration" ("Main Tab") T2."About" ("Main Tab") T2."Advance" ("Main Tab")] -> w1232
      frame "Home", Default {
      }
      frame "Test Setup" {
      }
      frame "Dashboard" {
      }
      frame "Imaging" {
      }
      frame "Report" {
      }
      frame "Analysis" {
      }
      frame "Calibration" {
      }
      frame "About" {
      }
      frame "Advance" {
      }
    }
    n1220 = Wait (ms)(milliseconds to wait=u32 100) -> ()  [unwired: 1 out]
    n1221 = local read "Main Tab Display"() -> (w1252:T4)
    n1222 = local write "Main Tab"(w1232) -> ()
    n1223 = case shown="\"Dashboard 3\"" w1252 {
      frame "Dashboard 1", Default {
        n1224 = property on="Reset Graph" class="Bool (strict)"("Visible"=FALSE) -> ()  [unwired: 2 in, 2 out]
      }
      frame "Dashboard 2" {
        n1225 = property on="Reset Graph" class="Bool (strict)"("Visible"=TRUE) -> ()  [unwired: 2 in, 2 out]
      }
      frame "Dashboard 3" {
        n1226 = property on="Reset Graph" class="Bool (strict)"("Visible"=TRUE) -> ()  [unwired: 2 in, 2 out]
      }
    }
    n1227 = local read "SCAR MEASURMENT"() -> (w1240:enum32{"Auto Scar", "Manual Scar"})
    n1228 = local read "Humidity"() -> (w1255:bool)
    n1229 = local read "Cap Live Image"() -> (w1237:bool)
    n1230 = local read "Sample Temperature"() -> (w1247:bool)
    n1231 = local read "Air Temp vs Humidity"() -> (w1245:bool)
    n1232 = local read "Frequency"() -> (w1246:bool)
    n1233 = case shown="True" w1255 {
      frame False {
        n1234 = local write "Humidity On Command"(TRUE ("Humidity On Command")) -> ()
        n1235 = case shown="True" "Humidity Off Command" {
          selector: "Humidity Off Command" -> [_ w1543]
          frame False {
          }
          frame True {
            n1236 = stacked-sequence {
              frame #0 {
                n1237 = local read "Write UNO"() -> (w1545:string[])
                n1238 = Insert Into Array(array=w1545, new element="R;1" ("new element/subarray")) -> (w1544:string[])  [unwired: 1 in]
                n1239 = local write "Write UNO"(w1544) -> ()
              }
              frame #1 {
                n1240 = Wait (ms)(milliseconds to wait=u32 2000) -> ()  [unwired: 1 out]
              }
              frame #2 {
                n1241 = local read "Write UNO"() -> (w1548:string[])
                n1242 = local read "EVENT LOG"() -> (w1552:string)
                n1243 = call "Event Log.vi"("Content"="Humidity Control Off" ("string"), "EVENT LOG"=w1552) -> ("EVENT LOG"=w1553:string)  [unwired: 8 in, 1 out]
                n1244 = local write "EVENT LOG"(w1553) -> ()
                n1245 = Insert Into Array(array=w1548, new element="R;1" ("new element/subarray")) -> (w1549:string[])  [unwired: 1 in]
                n1246 = local write "Write UNO"(w1549) -> ()
              }
            }
            n1247 = Not(x=w1543) -> (.not. x?=w1542:bool)
            n1248 = local write "Humidity Off Command"(w1542) -> ()
          }
        }
      }
      frame True {
        n1249 = local write "Humidity Off Command"(TRUE ("Humidity Off Command")) -> ()
        n1250 = case shown="True" "Humidity On Command" {
          selector: "Humidity On Command" -> [_ w1557]
          frame False {
          }
          frame True {
            n1251 = stacked-sequence {
              frame #0 {
                n1252 = local read "Set Rh"() -> (w1563:dbl)
                n1253 = local read "Write UNO"() -> (w1558:string[])
                n1254 = Number To Fractional String(number=w1563, precision (6)=i16 2) -> (F-format string=w1564:string)  [unwired: 2 in]
                n1255 = Concatenate Strings("M;" ("new element/subarray"), w1564) -> (w1562:string)
                n1256 = Insert Into Array(array=w1558, new element=w1562) -> (w1559:string[])  [unwired: 1 in]
                n1257 = local write "Write UNO"(w1559) -> ()
              }
              frame #1 {
                n1258 = Wait (ms)(milliseconds to wait=u32 2000) -> ()  [unwired: 1 out]
              }
              frame #2 {
                n1259 = local read "Set Rh"() -> (w1571:dbl)
                n1260 = local read "Write UNO"() -> (w1566:string[])
                n1261 = Number To Fractional String(number=w1571, precision (6)=i16 2) -> (F-format string=w1572:string)  [unwired: 2 in]
                n1262 = Concatenate Strings("M;" ("new element/subarray"), w1572) -> (w1570:string)
                n1263 = Insert Into Array(array=w1566, new element=w1570) -> (w1567:string[])  [unwired: 1 in]
                n1264 = local write "Write UNO"(w1567) -> ()
              }
              frame #3 {
                n1265 = Wait (ms)(milliseconds to wait=u32 1500) -> ()  [unwired: 1 out]
              }
              frame #4 {
                (unwired) "% RH" ("string")
                (unwired) i16 2 ("precision (6)")
                (unwired) "M;" ("new element/subarray")
                n1266 = local read "Set Rh"() -> (w1581:dbl)
                n1267 = local read "Write UNO"() -> (w1574:string[])
                n1268 = Number To Fractional String(number=w1581, precision (6)=i16 2) -> (F-format string=w1578:string)  [unwired: 2 in]
                n1269 = Concatenate Strings("M;" ("new element/subarray"), w1578) -> (w1582:string)
                n1270 = Concatenate Strings("Humidity Set to : " ("string"), w1578, "% RH" ("string")) -> (w1576:string)
                n1271 = Insert Into Array(array=w1574, new element=w1582) -> (w1575:string[])  [unwired: 1 in]
                n1272 = disable-structure shown="Enabled" {
                  frame Enabled {
                    n1273 = local read "EVENT LOG"() -> (w1585:string)
                    n1274 = call "Event Log.vi"("Content"="Humidity Control On", "EVENT LOG"=w1585) -> ("EVENT LOG"=w1586:string)  [unwired: 8 in, 1 out]
                    n1275 = local write "EVENT LOG"(w1586) -> ()
                  }
                  frame Disabled {
                  }
                }
                n1276 = disable-structure shown="Enabled" {
                  disable-tunnel: w1576 -> [_ _]
                  frame Enabled {
                    n1277 = local read "EVENT LOG"() -> (w1588:string)
                    n1278 = call "Event Log.vi"("Content"="Humidity Control On", "EVENT LOG"=w1588) -> ("EVENT LOG"=w1589:string)  [unwired: 8 in, 1 out]
                    n1279 = local write "EVENT LOG"(w1589) -> ()
                  }
                  frame Disabled {
                  }
                }
                n1280 = local write "Write UNO"(w1575) -> ()
              }
            }
            n1281 = Not(x=w1557) -> (.not. x?=w1556:bool)
            n1282 = local write "Humidity On Command"(w1556) -> ()
          }
        }
      }
    }
    n1283 = Equal?(x=w1240, y=enum32{"Auto Scar", "Manual Scar"}."Auto Scar" ("SCAR MEASURMENT")) -> (x = y?=w1236:bool)
    n1284 = local read "TEST STANDARD"() -> (w1243:T3)
    n1285 = And(x=w1237, y=w1236) -> (x .and. y?=w1238:bool)
    n1286 = case shown="True" w1238 {
      selector: w1238 -> [_ w1342]
      tunnel: errorcluster {"status"=FALSE, "code"=0, "source"=""} ("error in (no error) 3") -> [_ w1343]
      frame False {
      }
      frame True {
        n1287 = stacked-sequence {
          tunnel: w1343 -> [_ _ _ _ _ _ _ w1391]
          tunnel: w1342 -> [_ _ _ _ _ w1372 _ _]
          frame #0 {
            n1288 = call "CAMERA LIVE FEED FGV.vi"("Enum - Menu"=CAMERA_LIVE_FEED_ENUM."CAMERA MINIMIZE") -> ()  [unwired: 9 in, 2 out]
          }
          frame #1 {
            n1289 = property on="Auto Scar Check  2" class="Clust (strict)"("Visible"=TRUE) -> ()  [unwired: 2 in, 2 out]
          }
          frame #2 {
            n1290 = String To Path(string="C:\\LAB-IQ\\Image Calibrate v01.dcf") -> (path=w1348:path)
            n1291 = Open/Create/Replace File ("Open File")(file path (use dialog)=w1348) -> (refnum out=w1349:refnum<file>)  [unwired: 5 in, 2 out]
            n1292 = for {
              N: 4 -> [_]
              tunnel: w1349 -> [w1355]
              i -> [w1351]
              n1293 = Read from Text File ("Read File")(file (use dialog)=w1355) -> (text=w1356:string)  [unwired: 3 in, 3 out]
              n1294 = String Subset(string=w1356, offset (0)=6, length (rest)=10 ("length (rest)")) -> (substring=w1352:string)
              n1295 = Fract/Exp String To Number(string=w1352) -> (number=w1350:dbl)  [unwired: 3 in, 1 out]
              n1296 = case shown="0" w1351 {
                tunnel: w1350 -> [w1357 w1358 _ w1359 _]
                frame 0 {
                  "5x Gain" <- w1357
                }
                frame 1 {
                  "10x Gain" <- w1358
                }
                frame 2 {
                }
                frame 3 {
                  "100x gain" <- w1359
                }
                frame 4, Default {
                }
              }
            }
          }
          frame #3 {
            n1297 = local read "FILE 3"() -> (w1365:string)
            n1298 = call <vilib>:"Trim Whitespace.vi"("string"="C:\\LAB-IQ\\images\\") -> ("trimmed string"=w1367:string)  [unwired: 1 in]
            n1299 = String To Path(string=w1367) -> (path=w1366:path)
            n1300 = Concatenate Strings(w1365, ".png" ("string")) -> (w1364:string)
            n1301 = Build Path(base path=w1366, name or relative path=w1364) -> (appended path=w1362:path)
            "Image path" <- w1362
            n1302 = Path To String(path=w1362) -> (string=w1361:string)
            n1303 = call "CAMERA LIVE FEED FGV.vi"("Enum - Menu"=CAMERA_LIVE_FEED_ENUM."CAMERA SAVE", "Image Path"=w1361) -> ()  [unwired: 8 in, 2 out]
          }
          frame #4 {
            n1304 = One Button Dialog(message="Image saved successfully") -> ()  [unwired: 1 in, 1 out]
          }
          frame #5 {
            n1305 = local read "TEST STANDARD"() -> (w1371:T3)
            n1306 = local read "Magnification len live scar"() -> (w1383:string)
            n1307 = Not(x=w1372) -> (.not. x?=w1373:bool)
            n1308 = local write "Cap Live Image"(w1373) -> ()
            n1309 = case shown="\"ISO 12156\"" w1371 {
              tunnel: ["ASTM D6079" "ISO 12156"] -> w1370
              frame "ASTM D6079", Default {
              }
              frame "ISO 12156" {
              }
            }
            n1310 = case shown="\"5x\", Default" w1383 {
              tunnel: [w1386 w1387] -> w1382
              frame "5x", Default {
                n1311 = local read "5x Gain"() -> (w1386:dbl)
              }
              frame "10x" {
                # "5x"
                n1312 = local read "10x Gain"() -> (w1387:dbl)
              }
            }
            n1313 = local read "Image path"() -> (w1381:path)
            n1314 = local read "FILE 3"() -> (w1374:string)
            n1315 = call "EDGE DETCTION.vi"("GAIN VALUE"=w1382, "Image Path"=w1381) -> ("error out"=w1380:errorcluster, "return value"=w1379:cluster{string, string, dbl, dbl, dbl})  [unwired: 8 in]
            n1316 = Bundle By Name(cluster=T23 {"File Name"="", "Test Method"="", "Operator"="", "Fuel Description"="", "Date and time"=""} ("Main Ref"), "File Name"=w1374, "Test Method"=w1370) -> (w1375:T23)
            n1317 = call "duf file read.vi"("error in (no error)"=w1380, "Main Ref"=w1375) -> ("error out"=w1378:errorcluster, "Main Ref 2"=w1376:T23)  [unwired: 8 in]
            n1318 = call "EDGE DETECTION REPORT.vi"("error in (no error)"=w1378, "return value 2"=w1379, "Main Ref"=w1376) -> ()  [unwired: 8 in, 1 out]
          }
          frame #6 {
            n1319 = property on="Auto Scar Check  2" class="Clust (strict)"("Visible"=FALSE) -> ()  [unwired: 2 in, 2 out]
          }
          frame #7 {
            n1320 = call "CAMERA LIVE FEED FGV.vi"("Enum - Menu"=CAMERA_LIVE_FEED_ENUM."CAMERA MINIMIZE", "error in (no error)"=w1391) -> ()  [unwired: 8 in, 2 out]
            n1321 = local write "Main Dashboard Buttons"(T1."Home" ("Main Dashboard Buttons")) -> ()
            n1322 = local write "Main Tab"(T2."HOME" ("Main Tab")) -> ()
          }
        }
      }
    }
    n1323 = local read "Heater Button"() -> (w1244:bool)
    n1324 = case shown="True" w1246 {
      selector: w1246 -> [_ w1521]
      frame False {
      }
      frame True {
        n1325 = Not(x=w1521) -> (.not. x?=w1519:bool)
        n1326 = local write "Frequency"(w1519) -> ()
        n1327 = local write "Tab Control 2"(T6."Frequency" ("Tab Control 2")) -> ()
      }
    }
    n1328 = case shown="True" w1245 {
      selector: w1245 -> [_ w1518]
      frame False {
      }
      frame True {
        n1329 = Not(x=w1518) -> (.not. x?=w1516:bool)
        n1330 = local write "Air Temp vs Humidity"(w1516) -> ()
        n1331 = local write "Tab Control 2"(T6."Air Temp vs Rh" ("Tab Control 2")) -> ()
      }
    }
    n1332 = case shown="True" w1247 {
      selector: w1247 -> [_ w1524]
      frame False {
      }
      frame True {
        n1333 = Not(x=w1524) -> (.not. x?=w1522:bool)
        n1334 = local write "Sample Temperature"(w1522) -> ()
        n1335 = local write "Tab Control 2"(T6."Sample Temperature" ("Tab Control 2")) -> ()
      }
    }
    n1336 = case shown="\"Custom\"" w1243 {
      frame "ASTM D6079", Default {
        w1497 = "ASTM D6079 TEST CONDITIONS" ("Standard 2")
        n1337 = local write "Standard 2"(w1497) -> ()
        n1338 = local write "Standard"(w1497) -> ()
      }
      frame "ISO 12156" {
        w1498 = "ISO 12156 TEST CONDITIONS" ("Standard 2")
        n1339 = local write "Standard 2"(w1498) -> ()
        n1340 = local write "Standard"(w1498) -> ()
      }
      frame "CEC F-096-A-06" {
        w1499 = "CEC F-096-A-06 TEST CONDITIONS" ("Standard 2")
        n1341 = local write "Standard 2"(w1499) -> ()
        n1342 = local write "Standard"(w1499) -> ()
      }
      frame "Custom" {
        w1500 = "CUSTOM TEST CONDITIONS" ("Standard 2")
        n1343 = local write "Standard 2"(w1500) -> ()
        n1344 = local write "Standard"(w1500) -> ()
      }
    }
    n1345 = case shown="True" w1244 {
      frame False {
        n1346 = local write "Temperature On Command"(TRUE ("Temperature On Command")) -> ()
        n1347 = case shown="True" "Temperature Off Command" {
          selector: "Temperature Off Command" -> [_ w1504]
          frame False {
          }
          frame True {
            n1348 = Not(x=w1504) -> (.not. x?=w1503:bool)
            n1349 = local read "EVENT LOG"() -> (w1507:string)
            n1350 = local write "Temperature Off Command"(w1503) -> ()
            n1351 = call "Event Log.vi"("Content"="Heater Off", "EVENT LOG"=w1507) -> ("EVENT LOG"=w1506:string)  [unwired: 8 in, 1 out]
            n1352 = local write "EVENT LOG"(w1506) -> ()
          }
        }
      }
      frame True {
        n1353 = local write "Temperature Off Command"(TRUE ("Temperature Off Command")) -> ()
        n1354 = case shown="True" "Temperature On Command" {
          selector: "Temperature On Command" -> [_ w1511]
          frame False {
          }
          frame True {
            n1355 = Not(x=w1511) -> (.not. x?=w1510:bool)
            n1356 = local write "Temperature On Command"(w1510) -> ()
            n1357 = disable-structure shown="Enabled" {
              disable-tunnel: "Heater On" -> [w1513 _]
              frame Enabled {
                n1358 = local read "EVENT LOG"() -> (w1514:string)
                n1359 = call "Event Log.vi"("Content"=w1513, "EVENT LOG"=w1514) -> ("EVENT LOG"=w1515:string)  [unwired: 8 in, 1 out]
                n1360 = local write "EVENT LOG"(w1515) -> ()
              }
              frame Disabled {
              }
            }
          }
        }
      }
    }
    n1361 = local read "Main Tab"() -> (w1235:T2)
    n1362 = case shown="\"About\"" w1235 {
      frame "HOME", Default {
        w1278 = T17."Enabled" ("Disabled")
        n1363 = local read "Service Password enable"() -> (w1280:bool)
        n1364 = property on="Imaging" class="Bool (strict)"("DisabledEnum"=w1278) -> ()  [unwired: 2 in, 2 out]
        n1365 = property on="Dashboard" class="Bool (strict)"("DisabledEnum"=w1278) -> ()  [unwired: 2 in, 2 out]
        n1366 = property on="Test Setup" class="Bool (strict)"("DisabledEnum"=w1278) -> ()  [unwired: 2 in, 2 out]
        n1367 = property on="Analysis" class="Bool (strict)"("DisabledEnum"=w1278) -> ()  [unwired: 2 in, 2 out]
        n1368 = property on="Home" class="Bool (strict)"("DisabledEnum"=w1278) -> ()  [unwired: 2 in, 2 out]
        n1369 = property on="Report" class="Bool (strict)"("DisabledEnum"=w1278) -> ()  [unwired: 2 in, 2 out]
        n1370 = property on="Main Dashboard Buttons" class="RadioBtnsControl (strict)"("DisabledEnum"=w1278) -> ()  [unwired: 2 in, 2 out]
        n1371 = property on="Calibration" class="Bool (strict)"("DisabledEnum"=w1278) -> ()  [unwired: 2 in, 2 out]
        n1372 = case shown="True" w1280 {
          tunnel: [T17."Disabled" ("Disabled") T17."Enabled" ("Disabled")] -> w1279
          frame False {
          }
          frame True {
          }
        }
        n1373 = property on="About" class="Bool (strict)"("DisabledEnum"=w1279) -> ()  [unwired: 2 in, 2 out]
      }
      frame "Test Setup" {
        w1285 = T17."Enabled" ("Disabled")
        n1374 = local read "Service Password enable"() -> (w1284:bool)
        n1375 = property on="Dashboard" class="Bool (strict)"("DisabledEnum"=T17."Disabled" ("Disabled")) -> ()  [unwired: 2 in, 2 out]
        n1376 = property on="Imaging" class="Bool (strict)"("DisabledEnum"=w1285) -> ()  [unwired: 2 in, 2 out]
        n1377 = property on="Analysis" class="Bool (strict)"("DisabledEnum"=w1285) -> ()  [unwired: 2 in, 2 out]
        n1378 = property on="Home" class="Bool (strict)"("DisabledEnum"=w1285) -> ()  [unwired: 2 in, 2 out]
        n1379 = property on="Report" class="Bool (strict)"("DisabledEnum"=w1285) -> ()  [unwired: 2 in, 2 out]
        n1380 = property on="Test Setup" class="Bool (strict)"("DisabledEnum"=w1285) -> ()  [unwired: 2 in, 2 out]
        n1381 = case shown="True" w1284 {
          tunnel: [T17."Disabled" ("Disabled") T17."Enabled" ("Disabled")] -> w1283
          frame False {
          }
          frame True {
          }
        }
        n1382 = property on="About" class="Bool (strict)"("DisabledEnum"=w1283) -> ()  [unwired: 2 in, 2 out]
      }
      frame "Adv Scar" {
        w1292 = T17."Enabled" ("Disabled")
        n1383 = property on="Dashboard" class="Bool (strict)"("DisabledEnum"=T17."Disabled" ("Disabled")) -> ()  [unwired: 2 in, 2 out]
        n1384 = property on="Imaging" class="Bool (strict)"("DisabledEnum"=w1292) -> ()  [unwired: 2 in, 2 out]
        n1385 = property on="Analysis" class="Bool (strict)"("DisabledEnum"=w1292) -> ()  [unwired: 2 in, 2 out]
        n1386 = property on="Home" class="Bool (strict)"("DisabledEnum"=w1292) -> ()  [unwired: 2 in, 2 out]
        n1387 = property on="Report" class="Bool (strict)"("DisabledEnum"=w1292) -> ()  [unwired: 2 in, 2 out]
        n1388 = property on="Test Setup" class="Bool (strict)"("DisabledEnum"=w1292) -> ()  [unwired: 2 in, 2 out]
        n1389 = local read "Service Password enable"() -> (w1290:bool)
        n1390 = case shown="True" w1290 {
          tunnel: [T17."Disabled" ("Disabled") T17."Enabled" ("Disabled")] -> w1289
          frame False {
          }
          frame True {
          }
        }
        n1391 = property on="About" class="Bool (strict)"("DisabledEnum"=w1289) -> ()  [unwired: 2 in, 2 out]
      }
      frame "Calibration" {
        w1295 = T17."Enabled" ("Disabled")
        n1392 = property on="Dashboard" class="Bool (strict)"("DisabledEnum"=T17."Disabled" ("Disabled")) -> ()  [unwired: 2 in, 2 out]
        n1393 = property on="Imaging" class="Bool (strict)"("DisabledEnum"=w1295) -> ()  [unwired: 2 in, 2 out]
        n1394 = property on="Analysis" class="Bool (strict)"("DisabledEnum"=w1295) -> ()  [unwired: 2 in, 2 out]
        n1395 = property on="Home" class="Bool (strict)"("DisabledEnum"=w1295) -> ()  [unwired: 2 in, 2 out]
        n1396 = property on="Report" class="Bool (strict)"("DisabledEnum"=w1295) -> ()  [unwired: 2 in, 2 out]
        n1397 = property on="Test Setup" class="Bool (strict)"("DisabledEnum"=w1295) -> ()  [unwired: 2 in, 2 out]
        n1398 = local read "Service Password enable"() -> (w1297:bool)
        n1399 = property on="Calibration" class="Bool (strict)"("DisabledEnum"=w1295) -> ()  [unwired: 2 in, 2 out]
        n1400 = case shown="True" w1297 {
          tunnel: [T17."Disabled" ("Disabled") T17."Enabled" ("Disabled")] -> w1296
          frame False {
          }
          frame True {
          }
        }
        n1401 = property on="About" class="Bool (strict)"("DisabledEnum"=w1296) -> ()  [unwired: 2 in, 2 out]
      }
      frame "Adv Scar Report" {
        w1303 = T17."Enabled" ("Disabled")
        n1402 = property on="Dashboard" class="Bool (strict)"("DisabledEnum"=T17."Disabled" ("Disabled")) -> ()  [unwired: 2 in, 2 out]
        n1403 = property on="Imaging" class="Bool (strict)"("DisabledEnum"=w1303) -> ()  [unwired: 2 in, 2 out]
        n1404 = property on="Analysis" class="Bool (strict)"("DisabledEnum"=w1303) -> ()  [unwired: 2 in, 2 out]
        n1405 = property on="Home" class="Bool (strict)"("DisabledEnum"=w1303) -> ()  [unwired: 2 in, 2 out]
        n1406 = property on="Report" class="Bool (strict)"("DisabledEnum"=w1303) -> ()  [unwired: 2 in, 2 out]
        n1407 = property on="Test Setup" class="Bool (strict)"("DisabledEnum"=w1303) -> ()  [unwired: 2 in, 2 out]
        n1408 = local read "Service Password enable"() -> (w1302:bool)
        n1409 = case shown="True" w1302 {
          tunnel: [T17."Disabled" ("Disabled") T17."Enabled" ("Disabled")] -> w1301
          frame False {
          }
          frame True {
          }
        }
        n1410 = property on="About" class="Bool (strict)"("DisabledEnum"=w1301) -> ()  [unwired: 2 in, 2 out]
      }
      frame "Compare Files" {
        w1309 = T17."Enabled" ("Disabled")
        n1411 = local read "Service Password enable"() -> (w1308:bool)
        n1412 = property on="Dashboard" class="Bool (strict)"("DisabledEnum"=T17."Disabled" ("Disabled")) -> ()  [unwired: 2 in, 2 out]
        n1413 = property on="Imaging" class="Bool (strict)"("DisabledEnum"=w1309) -> ()  [unwired: 2 in, 2 out]
        n1414 = property on="Analysis" class="Bool (strict)"("DisabledEnum"=w1309) -> ()  [unwired: 2 in, 2 out]
        n1415 = property on="Home" class="Bool (strict)"("DisabledEnum"=w1309) -> ()  [unwired: 2 in, 2 out]
        n1416 = property on="Report" class="Bool (strict)"("DisabledEnum"=w1309) -> ()  [unwired: 2 in, 2 out]
        n1417 = property on="Test Setup" class="Bool (strict)"("DisabledEnum"=w1309) -> ()  [unwired: 2 in, 2 out]
        n1418 = case shown="True" w1308 {
          tunnel: [T17."Disabled" ("Disabled") T17."Enabled" ("Disabled")] -> w1307
          frame False {
          }
          frame True {
          }
        }
        n1419 = property on="About" class="Bool (strict)"("DisabledEnum"=w1307) -> ()  [unwired: 2 in, 2 out]
      }
      frame "Acquire" {
        n1420 = local read "Service Password enable"() -> (w1314:bool)
        n1421 = property on="Test Setup" class="Bool (strict)"("DisabledEnum"=T17."Disabled" ("Disabled")) -> ()  [unwired: 2 in, 2 out]
        n1422 = local read "Auto Start Test"() -> (w1316:bool)
        n1423 = local read "RUN"() -> (w1318:bool)
        n1424 = case shown="True" w1314 {
          tunnel: [T17."Disabled" ("Disabled") T17."Enabled" ("Disabled")] -> w1315
          frame False {
          }
          frame True {
          }
        }
        n1425 = Or(x=w1318, y=w1316) -> (x .or. y?=w1317:bool)
        n1426 = case shown="True" w1317 {
          tunnel: [T17."Enabled" ("Disabled") T17."Disabled" ("Disabled")] -> w1313
          frame False {
          }
          frame True {
          }
        }
        n1427 = property on="About" class="Bool (strict)"("DisabledEnum"=w1315) -> ()  [unwired: 2 in, 2 out]
        n1428 = property on="Imaging" class="Bool (strict)"("DisabledEnum"=w1313) -> ()  [unwired: 2 in, 2 out]
        n1429 = property on="Dashboard" class="Bool (strict)"("DisabledEnum"=w1313) -> ()  [unwired: 2 in, 2 out]
        n1430 = property on="Analysis" class="Bool (strict)"("DisabledEnum"=w1313) -> ()  [unwired: 2 in, 2 out]
        n1431 = property on="Home" class="Bool (strict)"("DisabledEnum"=w1313) -> ()  [unwired: 2 in, 2 out]
        n1432 = property on="Report" class="Bool (strict)"("DisabledEnum"=w1313) -> ()  [unwired: 2 in, 2 out]
        n1433 = property on="Calibration" class="Bool (strict)"("DisabledEnum"=w1313) -> ()  [unwired: 2 in, 2 out]
      }
      frame "About" {
        n1434 = local read "FILE"() -> (w1332:string)
        n1435 = local read "TEST FILE NAM,E SAVED"() -> (w1325:bool)
        n1436 = call <vilib>:"Trim Whitespace.vi"("string"=w1332) -> ("trimmed string"=w1331:string)  [unwired: 1 in]
        n1437 = local read "Auto Start Test"() -> (w1335:bool)
        n1438 = String Length(string=w1331) -> (length=w1330:i32)
        n1439 = Greater?(x=w1330, y=1) -> (0:w1327:bool)
        n1440 = And(x=w1327, y=w1325) -> (x .and. y?=w1326:bool)
        n1441 = local read "RUN"() -> (w1337:bool)
        n1442 = case shown="True" w1326 {
          tunnel: [T17."Disabled" ("Disabled") T17."Enabled" ("Disabled")] -> w1328
          frame False {
          }
          frame True {
          }
        }
        n1443 = Or(x=w1337, y=w1335) -> (x .or. y?=w1336:bool)
        n1444 = property on="About" class="Bool (strict)"("DisabledEnum"=T17."Enabled" ("Disabled")) -> ()  [unwired: 2 in, 2 out]
        n1445 = case shown="False" w1336 {
          tunnel: [T17."Enabled" ("Disabled") T17."Disabled" ("Disabled")] -> w1334
          frame False {
          }
          frame True {
          }
        }
        n1446 = property on="Dashboard" class="Bool (strict)"("DisabledEnum"=w1328) -> ()  [unwired: 2 in, 2 out]
        n1447 = property on="Test Setup" class="Bool (strict)"("DisabledEnum"=T17."Disabled" ("Disabled")) -> ()  [unwired: 2 in, 2 out]
        n1448 = property on="Imaging" class="Bool (strict)"("DisabledEnum"=w1334) -> ()  [unwired: 2 in, 2 out]
        n1449 = property on="Analysis" class="Bool (strict)"("DisabledEnum"=w1334) -> ()  [unwired: 2 in, 2 out]
        n1450 = property on="Home" class="Bool (strict)"("DisabledEnum"=w1334) -> ()  [unwired: 2 in, 2 out]
        n1451 = property on="Report" class="Bool (strict)"("DisabledEnum"=w1334) -> ()  [unwired: 2 in, 2 out]
      }
    }
    n1452 = local read "Quit"() -> (w1262:bool)
    "Single" <- "Single - Graph"
  }
  n1453 = disable-structure shown="Disabled" {
    disable-tunnel: [w1614 _] -> w43
    disable-tunnel: _ -> [w1613 _]
    frame Disabled {
      n1454 = while {
        tunnel: w1613 -> [_]
        tunnel: [w1615] -> w1614
        tunnel: [w1616] -> _
        i -> [w1616]
        stop <- w1615 stop-if-true
        w1632 = u16 10 items=["1.0"=10, "1.5"=15, "2.0"=20] ("stop bits (10: 1 bit)")
        n1455 = Wait (ms)(milliseconds to wait=u32 10) -> ()  [unwired: 1 out]
        n1456 = call-poly "VISA Configure Serial Port"("VISA resource name"=refnum<visa-resource-name> "ASRL1::INSTR" ("COM PORT"), "timeout (10sec)"=u32 10, "baud rate (9600)"=u32 57600, "data bits (8)"=u16 8, "stop bits (10: 1 bit)"=w1632) -> ("VISA resource name out"=w1618:refnum<visa-resource-name>, "error out"=w1627:errorcluster)  [unwired: 9 in]
        n1457 = VISA Read(VISA resource name=w1618, byte count=u32 2 ("byte count (0)")) -> (read buffer=w1626:string)  [unwired: 1 in, 3 out]
        n1458 = String Subset(string=w1626, offset (0)=0, length (rest)=2 ("length (rest)")) -> (substring=w1625:string)
        n1459 = Match Pattern(string=w1625, regular expression="<>") -> (offset past match=w1622:i32)  [unwired: 1 in, 3 out]
        n1460 = Greater Or Equal?(x=w1622, y=0) -> (x >= y?=w1617:bool)
        n1461 = case shown="True" w1617 {
          tunnel: w1618 -> [_ w1636]
          tunnel: w1627 -> [_ w1635]
          frame False {
          }
          frame True {
            n1462 = VISA Read(VISA resource name=w1636, byte count=u32 32 ("byte count (0)"), error in (no error)=w1635) -> (read buffer=w1634:string)  [unwired: 3 out]
            n1463 = String Subset(string=w1634, offset (0)=0, length (rest)=8 ("length (rest)")) -> (substring=w1638:string)
            n1464 = String Subset(string=w1634, offset (0)=8, length (rest)=8 ("length (rest)")) -> (substring=w1639:string)
            n1465 = Decimal String To Number(string=w1639) -> (number=w1646:i32)  [unwired: 2 in, 1 out]
            n1466 = Decimal String To Number(string=w1638) -> (number=w1642:i32)  [unwired: 2 in, 1 out]
            n1467 = Divide(x=w1646, y=10000) -> ()  [unwired: 1 out]
            n1468 = Divide(x=w1642, y=1000000) -> ()  [unwired: 1 out]
          }
        }
        n1469 = local read "Quit"() -> (w1615:bool)
      }
    }
    frame Enabled {
    }
  }
  n1470 = Tick Count (ms)() -> (millisecond timer value=w4:u32)
  n1471 = while {
    shift-right: [w1692] -> _
    shift-left: w6 -> [w1696]
    shift-right: [w1691] -> _
    shift-left: w5 -> [w1695]
    shift-right: [w1690] -> _
    shift-left: w6 -> [w1694]
    shift-right: [w1689] -> _
    shift-left: w5 -> [w1693]
    shift-right: [w1687] -> _
    shift-left: w4 -> [w1688]
    shift-right: [w1684] -> _
    shift-left: w3 -> [w1685]
    shift-right: [w1683] -> _
    shift-left: w3 -> [w1686]
    shift-right: [w1676] -> _
    shift-left: w3 -> [w1682]
    shift-right: [w1675] -> _
    shift-left: w3 -> [w1681]
    shift-right: [w1674] -> _
    shift-left: w3 -> [w1680]
    shift-right: [w1673] -> _
    shift-left: w3 -> [w1679]
    shift-right: [w1672] -> _
    shift-left: w3 -> [w1678]
    shift-right: [w1671] -> _
    shift-left: w3 -> [w1677]
    shift-right: [w1670] -> _
